vi "Navigation_Main_derping_stuff_up.vi"() -> ()   [LabVIEW 2015]
uses:
  <vilib>/myRIO/Instrument Drivers/Onboard IO/PWM/typedefs/PWM Reference.ctl
  <vilib>/myRIO/Common/Instrument Driver Framework/Utilities/typedefs/myRIO Generic Hardware Reference.ctl
  <vilib>/myRIO/Common/Instrument Driver Framework/Utilities/typedefs/Hardware Version Enum.ctl
  <vilib>/myRIO/Common/Instrument Driver Framework/Utilities/typedefs/myRIO v1.0 Reference.ctl
  <vilib>/myRIO/Common/Instrument Driver Framework/Utilities/typedefs/Generic FPGA Reference.ctl
  <vilib>/myRIO/Common/Instrument Driver Framework/myRIO v1.0/PWM/typedefs/PWM Channels Enum.ctl
  <vilib>/myRIO/Instrument Drivers/Onboard IO/PWM/typedefs/PWM Configuration.ctl
  <vilib>/userdefined/High Color/nirio_resource_hc.ctl
  <vilib>/myRIO/Common/Instrument Driver Framework/myRIO v1.0/PWM/vis/myRIO v1.1 Open PWM.vi
  <vilib>/myRIO/Common/Instrument Driver Framework/Utilities/vis/Validate Channels.vi
  <vilib>/myRIO/Common/Instrument Driver Framework/myRIO v1.0/PWM/vis/myRIO v1.0 Reserve PWM.vi
  <vilib>/myRIO/Common/Instrument Driver Framework/myRIO v1.0/PWM/vis/myRIO v1.0 Build MUX Configuration PWM.vi
  <vilib>/myRIO/Common/Instrument Driver Framework/myRIO v1.0/Resource Manager/vis/myRIO v1.0 Reserve Channel List.vi
  <vilib>/myRIO/Common/Instrument Driver Framework/myRIO v1.0/Resource Manager/vis/myRIO v1.0 Create Configuration List.vi
  <vilib>/myRIO/Common/Instrument Driver Framework/myRIO v1.0/Resource Manager/vis/myRIO v1.0 Reserve Channel.vi
  <vilib>/myRIO/Common/Instrument Driver Framework/myRIO v1.0/Resource Manager/vis/myRIO v1.0 Unreserve Channel.vi
  <vilib>/myRIO/Common/Instrument Driver Framework/myRIO v1.0/Resource Manager/vis/myRIO v1.0 Build Mutex Name.vi
  <vilib>/FPGAPlugInAG/myRIO-1900/niLvFpga_Open_myRIO-1900.vi
  <vilib>/rvi/interface/common/dynamic/niFpgaDynamicAddResources.vi
  <vilib>/myRIO/Common/Instrument Driver Framework/Utilities/vis/FPGA Ref Manager.vi
  <vilib>/Utility/error.llb/Error Cluster From Error Code.vi
  <vilib>/myRIO/Common/Instrument Driver Framework/Utilities/vis/Ref Counter.vi
  <vilib>/rvi/errors/niLvFpgaAdjustHostInterfaceError.vi
  <vilib>/Utility/VariantDataType/GetNumericInfo.vi
  <vilib>/myRIO/Common/Instrument Driver Framework/myRIO v1.0/myRIO v1.1 Open.vi
  <vilib>/myRIO/Common/Instrument Driver Framework/Utilities/vis/IO Manager.vi
  <vilib>/myRIO/Common/Instrument Driver Framework/Utilities/vis/Configuration Manager.vi
  <vilib>/myRIO/Common/Instrument Driver Framework/myRIO v1.0/Resource Manager/vis/myRIO v1.0 Configure IO.vi
  <vilib>/myRIO/Common/Instrument Driver Framework/myRIO v1.0/myRIO v1.0 Close.vi
  <vilib>/myRIO/Common/Instrument Driver Framework/myRIO v1.0/PWM/vis/myRIO v1.0 Write PWM.vi
  <vilib>/addons/control/pid/pid.llb/PID (DBL).vi
  <vilib>/rvi/interface/nirviOpenFPGA/nirviOpenFPGA.xnode
  Navi/E/FPGA Bitfiles/NavigationProjec_FPGATarget2_FPGAMainNavigati_PWPHW8gwDxI.lvbitx
  <vilib>/rvi/interface/nirviReadWriteControl/nirviReadWriteControl.xnode
  <vilib>/myRIO/Instrument Drivers/Onboard IO/PWM/vis/myRIO PWM Open.xnode
  <vilib>/myRIO/Instrument Drivers/Onboard IO/PWM/PWM.lvlib
  <vilib>/myRIO/Instrument Drivers/Utilities/Utilities.lvlib
  NiFpgaLv.dll
  <vilib>/rvi/interface/Simulation/niFpgaSimulationCallBeginRW.vi
  <vilib>/addons/control/pid/NI_PID_pid.lvlib
panel:
  out "goal reached":bool=TRUE
  out "x/y":dbl
  out "scale":dbl=1.0
  in  "x goal":dbl=10.0
  in  "L Desired Input Velocity (ft/s) 4":dbl(knob) scale=-4.0..4.0
  out "x position 5":dbl
  in  "R Min Linear Velocity (ft/s)  2":dbl=-2.0 format="%#_13g"
  in  "L Min Linear Velocity (ft/s) 9":dbl=-2.0 format="%#_13g"
  in  "R Max Linear Velocity (ft/s) 5":dbl=2.0 format="%#_13g"
  in  "L Max Linear Velocity (ft/s) 5":dbl=2.0 format="%#_13g"
  in  "R Desired Input Velocity (ft/s) 5":dbl(knob) scale=-4.0..4.0
  in  "R Desired Input Velocity (ft/s) 4":dbl(knob) scale=-4.0..4.0
  in  "L Desired Input Velocity (ft/s) 3":dbl(knob) scale=-4.0..4.0
  in  "R Desired Input Velocity (ft/s) 3":dbl(knob) scale=-4.0..4.0
  in  "L Desired Input Velocity (ft/s) 2":dbl(knob) scale=-4.0..4.0
  in  "R Desired Input Velocity (ft/s) 2":dbl(knob) scale=-4.0..4.0
  in  "L Desired Input Velocity (ft/s)":dbl(knob) scale=-4.0..4.0
  out "left":dbl
  out "right":dbl
  out "actual pwm 2":dbl
  in  "stop 3":bool
  out "left pwm":dbl(graph)
  out "dt out (s) 3":dbl format="%.3f"
  in  "output range 3":cluster{"output high":dbl, "output low":dbl}={"output high"=0.13333, "output low"=-0.13333} {"output low" format="%.6f"; "output high" format="%.5f"}
  in  "PID gains 3":T1={"proportional gain (Kc)"=0.002, "integral time (Ti, min)"=7e-07, "derivative time (Td, min)"=0.0} {"derivative time (Td, min)" format="%.8f"; "integral time (Ti, min)" format="%.8f"; "proportional gain (Kc)" format="%.8f"}
  out "desired pwm 2":dbl
  out "feedback 2":dbl
  out ".not. x? 3":bool
  out "Elapsed Time (s) 2":dbl caption="Elapsed Time (s)"
  out "x traveled 2":dbl
  out "y traveled 2":dbl
  out "avg 124":dbl
  out "avg 457":dbl
  out "psi dot 2":dbl
  out "distance traveled 2":dbl
  out "y dot 2":dbl
  out "x dot 2":dbl
  out "x position 2":dbl
  out "y position 2":dbl
  out "reset x y 2":dbl
  out "Tick Count(mSec) 2":u32 caption="Tick Count(mSec)"
  in  "start y 2":dbl=3.0
  in  "start x 2":dbl=1.0
  in  "Encoder Reset 3":bool
  out "ENC.B_c.CNTR 3":i32
  out "ENC.B_b.CNTR 3":i32
  out "ENC.B_a.CNTR 3":i32
  out "ENC.A_c.CNTR 3":i32
  out "ENC.A_b.CNTR 3":i32
  out "ENC.A_a.CNTR 3":i32
  in  "start y":dbl=3.0
  in  "start x":dbl=1.0
  in  "Encoder Reset 2":bool
  out "actual pwm":dbl
  in  "stop 2":bool
  out "right pwm":dbl(graph)
  out "dt out (s) 2":dbl format="%.3f"
  in  "output range 2":cluster{"output high":dbl, "output low":dbl}={"output high"=0.13333, "output low"=-0.13333} {"output low" format="%.6f"; "output high" format="%.5f"}
  in  "PID gains 2":T1={"proportional gain (Kc)"=0.002, "integral time (Ti, min)"=7e-07, "derivative time (Td, min)"=0.0} {"derivative time (Td, min)" format="%.8f"; "integral time (Ti, min)" format="%.8f"; "proportional gain (Kc)" format="%.8f"}
  out "desired pwm":dbl
  out "feedback":dbl
  out ".not. x? 2":bool
  out "Elapsed Time (s)":dbl
  out "LF Rot Velocity (rot/s)":dbl
  out "LM Rot Velocity (rot/s)":dbl
  out "LR Rot Velocity (rot/s)":dbl
  out "RR Rot Velocity (rot/s)":dbl
  out "RM Linear Velocity (rot/s)":dbl
  out "RF Linear Velocity (rot/s)":dbl
  in  "Encoder Reset":bool
  out "SYS.SELECTA":u8 format="%08b"
  out "ENC.B_c.CNTR":i32
  out "ENC.B_b.CNTR":i32
  out "ENC.B_a.CNTR":i32
  out "ENC.A_c.CNTR":i32
  out "ENC.A_b.CNTR":i32
  out "ENC.A_a.CNTR":i32
  in  "R Min Linear Velocity (ft/s)":dbl=-2.0 format="%#_13g"
  in  "R Max Linear Velocity (ft/s)":dbl=2.0 format="%#_13g"
  in  "L Min Linear Velocity (ft/s)":dbl=-2.0 format="%#_13g"
  in  "L Max Linear Velocity (ft/s)":dbl=2.0 format="%#_13g"
  out "Current Rot Velocity (rot/s)":T2(graph)
  # "Motor Control Parameters"
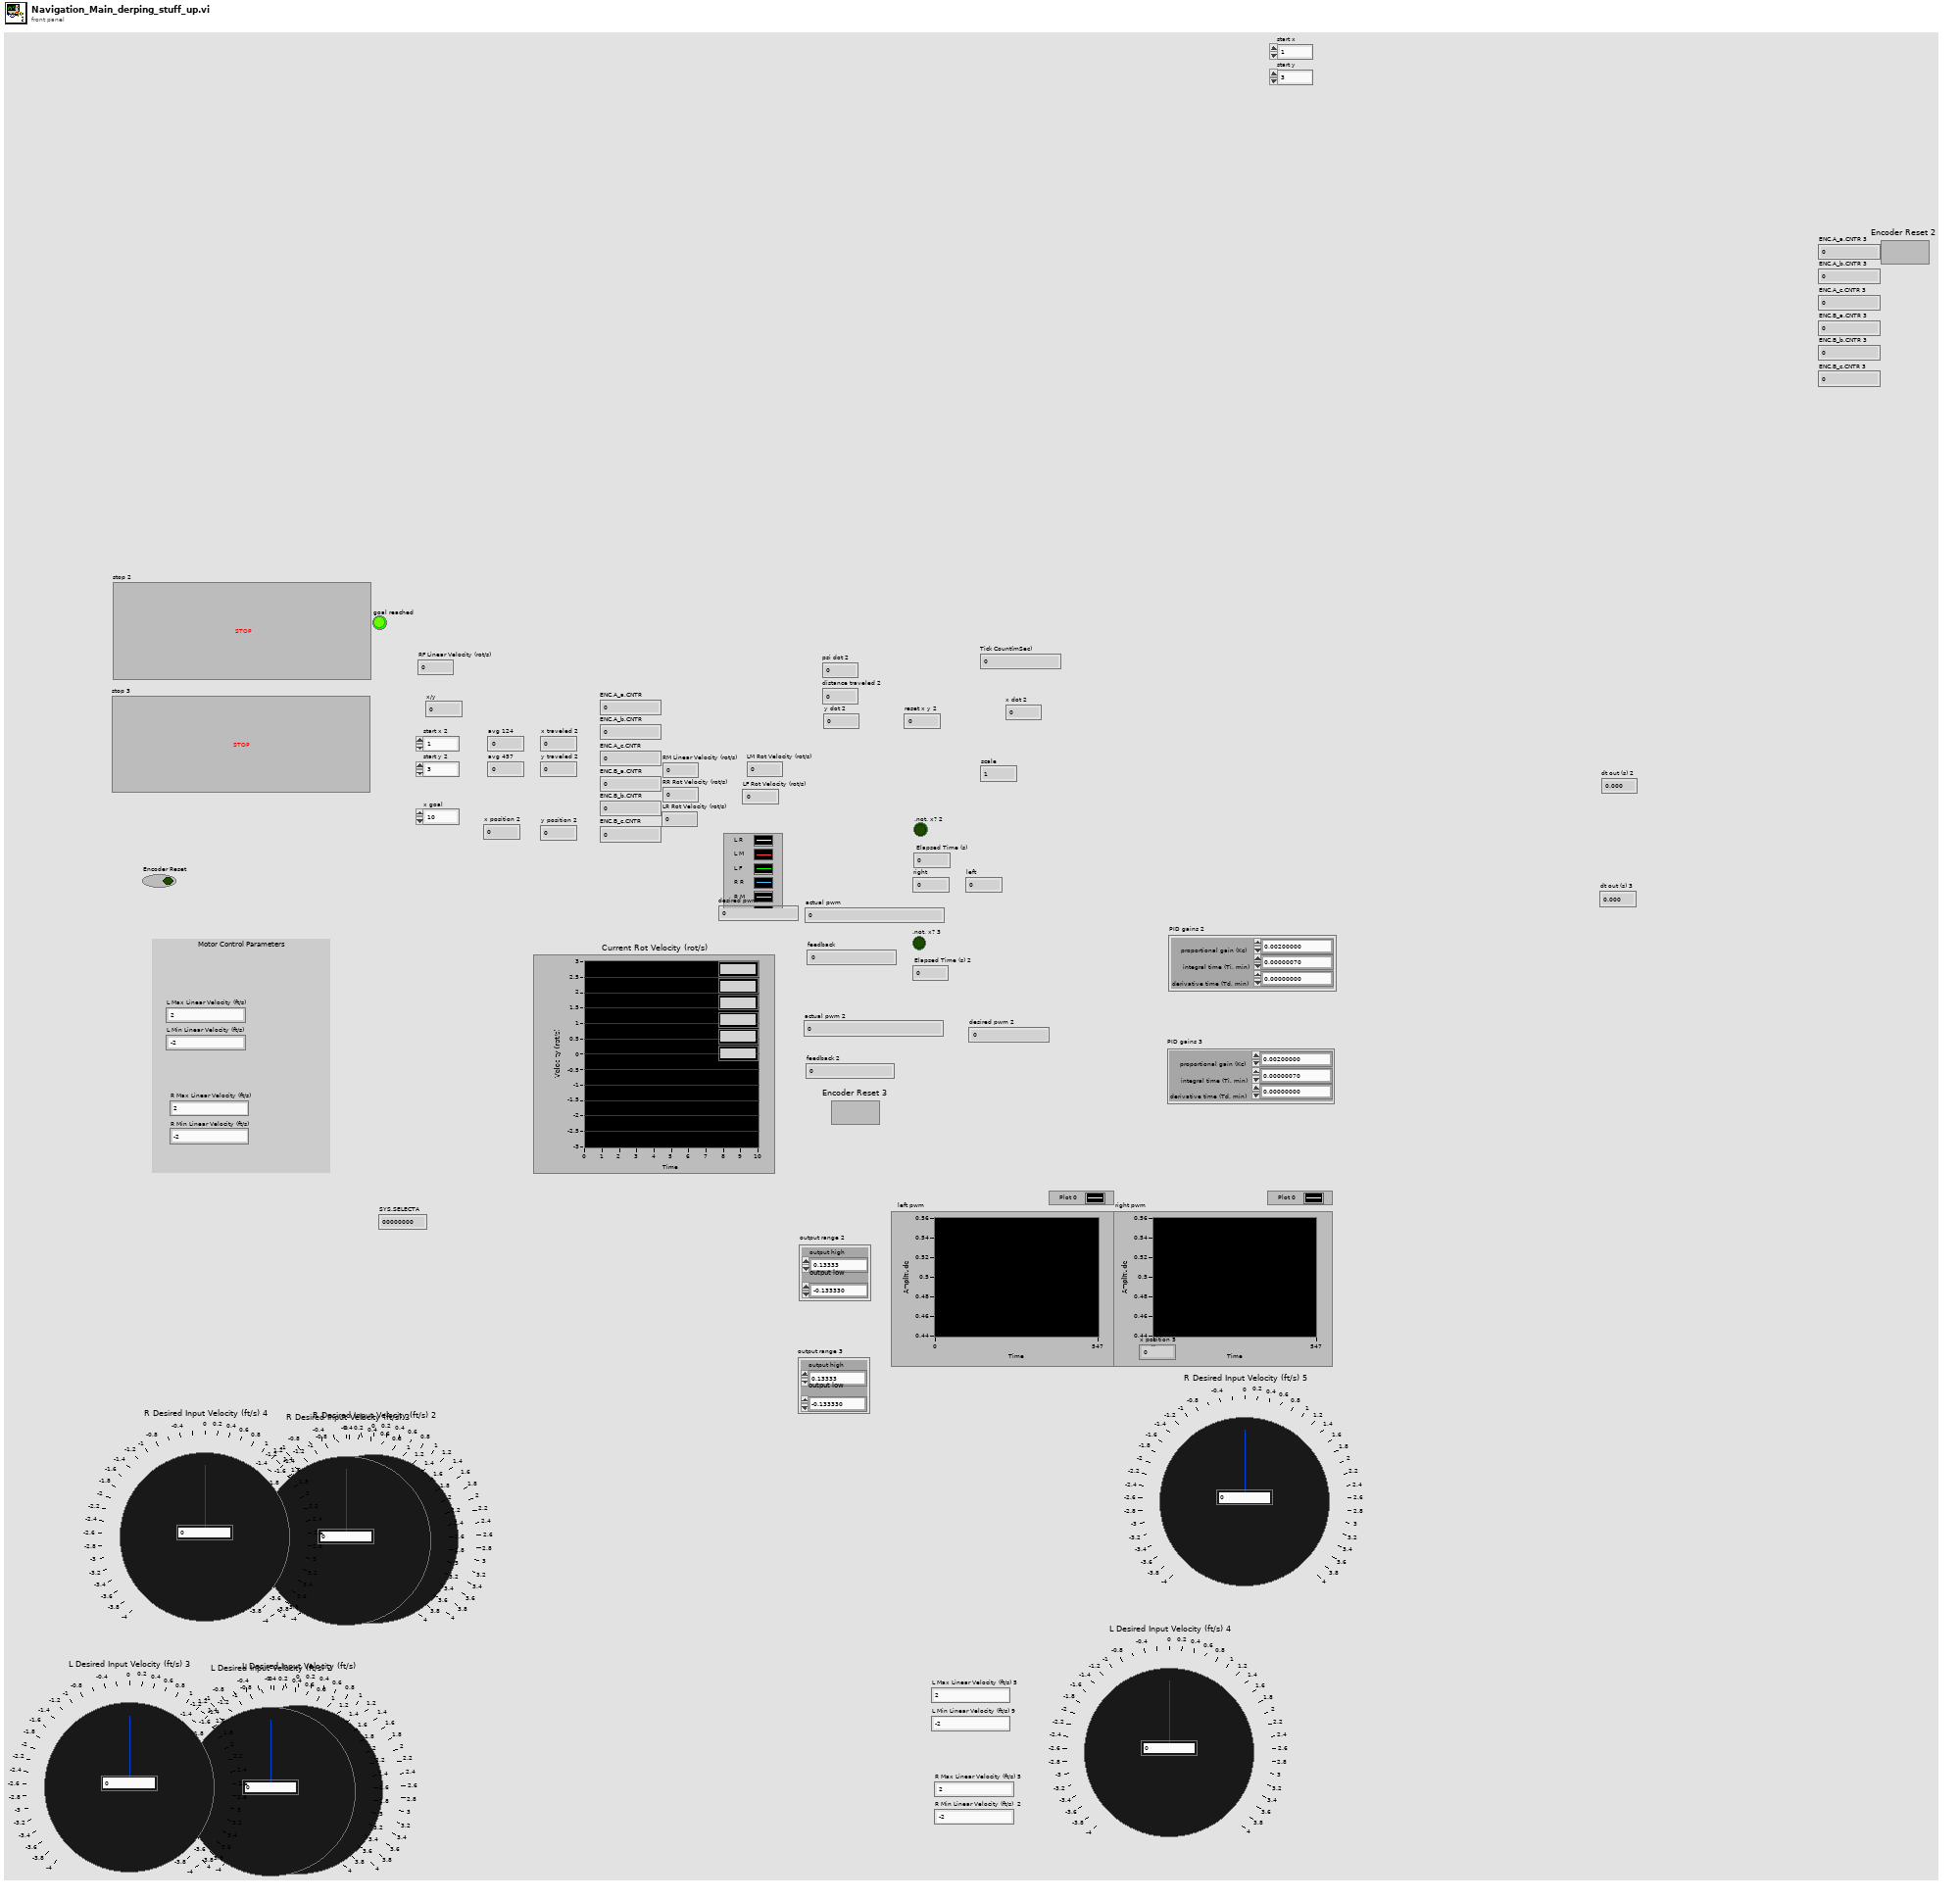
[diagram p1: front panel]
types:
  T1 = cluster{"proportional gain (Kc)":dbl, "integral time (Ti, min)":dbl, "derivative time (Td, min)":dbl}
  T2 = cluster{"Rotational Velocity (RPS)":dbl, "Rotational Velocity (RPS)":dbl, "Rotational Velocity (RPS)":dbl, "Rotational Velocity (RPS)":dbl, "Rotational Velocity (RPS)":dbl, "Rotational Velocity (RPS)":dbl}
  T3 = typedef "nirio_resource_hc.ctl" = tag
  T4 = typedef "Hardware Version Enum.ctl" = enum16{"Unknown", "myRIO-1900", "myRIO-1950", "roboRIO"}
  T5 = typedef "PWM.lvlib/PWM Reference.ctl" = cluster{"myRIO Reference":T6, "PWM Channels Enum":T9, "PWM Configuration":T10}
  T6 = typedef "myRIO Generic Hardware Reference.ctl" = cluster{"myRIO Model":T4, "myRIO Hardware Reference":T7}
  T7 = typedef "myRIO v1.0 Reference.ctl" = cluster{"Generic FPGA Reference":T8, "Allow multiple opens":bool}
  T8 = typedef "Generic FPGA Reference.ctl" = refnum<k20>
  T9 = typedef "PWM Channels Enum.ctl" = enum16{"Not Connected", "C/PWM0", "C/PWM1", "A/PWM0", "A/PWM1", "A/PWM2", "B/PWM0", "B/PWM1", "B/PWM2", "PWM/PWM0", "PWM/PWM1", "PWM/PWM2", "PWM/PWM3", "PWM/PWM4", "PWM/PWM5", "PWM/PWM6", "PWM/PWM7", "PWM/PWM8", "PWM/PWM9"}
  T10 = typedef "PWM.lvlib/PWM Configuration.ctl" = cluster{"Frequency":dbl, "Duty Cycle":dbl}
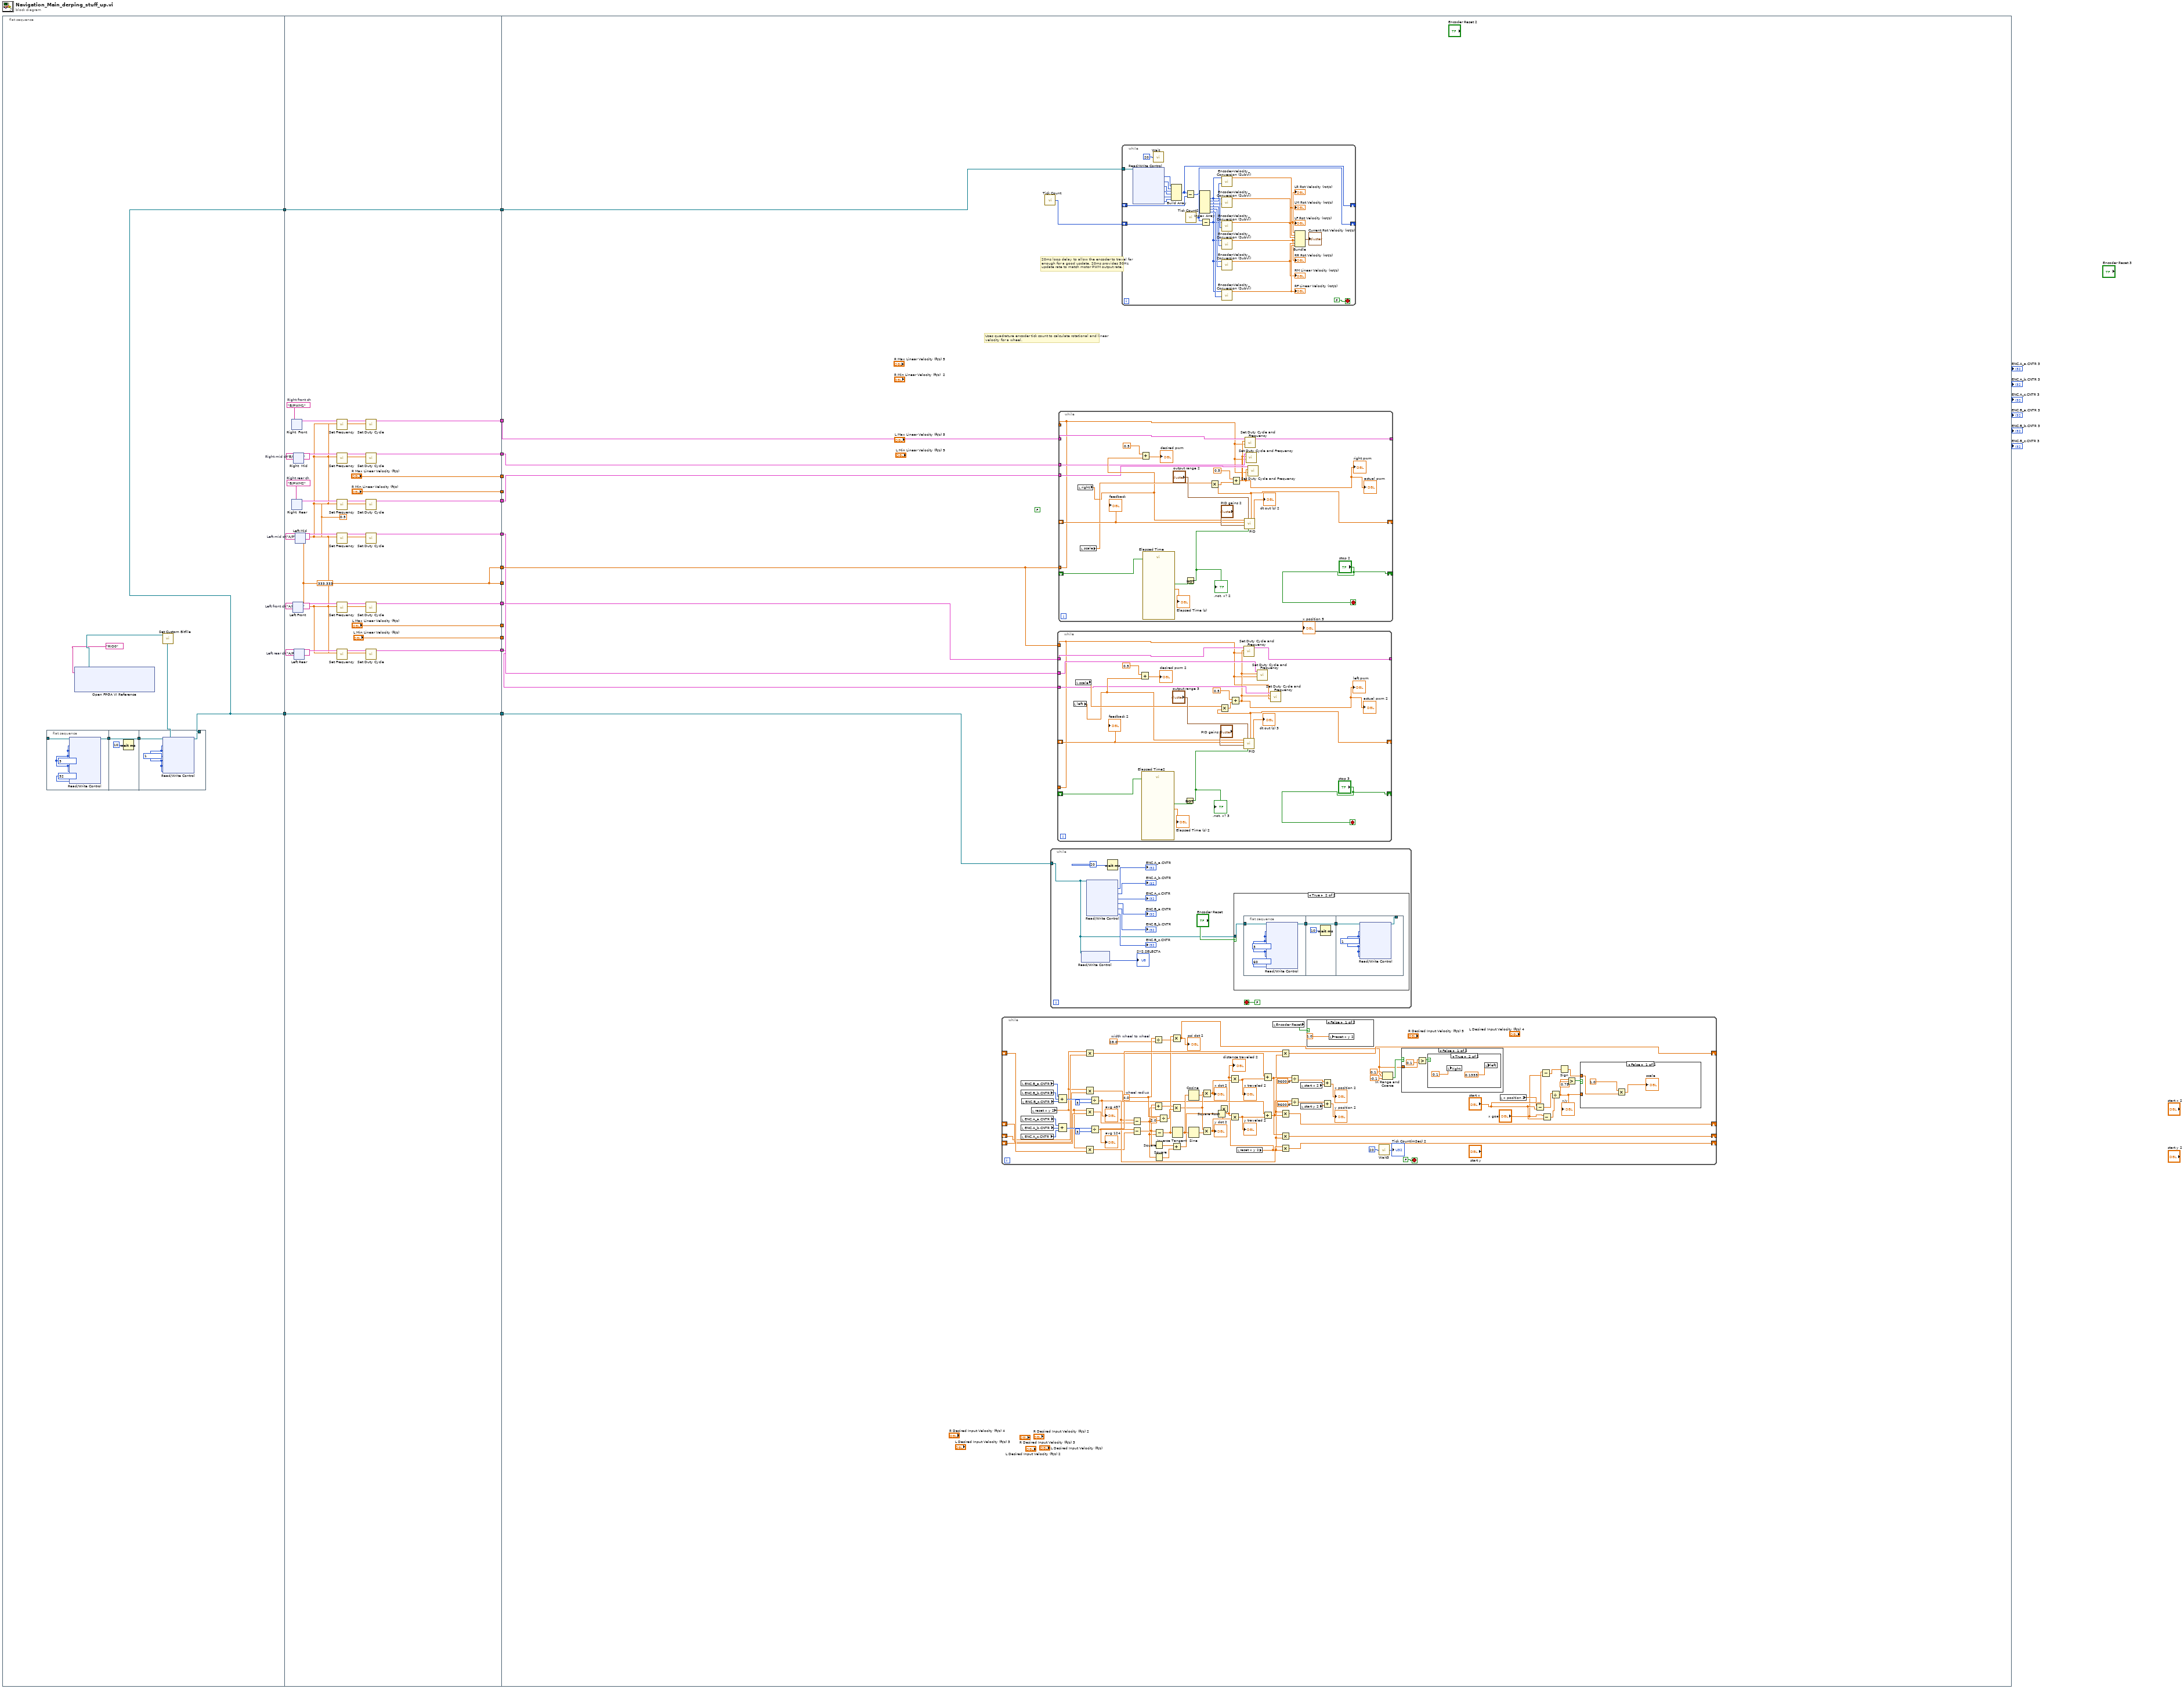
[diagram p0: block diagram]
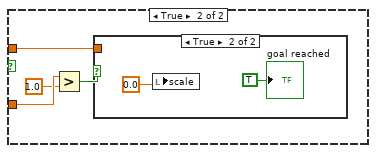
[diagram p2: hidden frame]
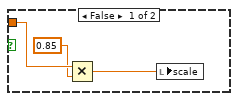
[diagram p3: hidden frame]
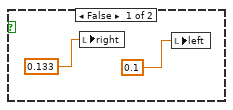
[diagram p4: hidden frame]
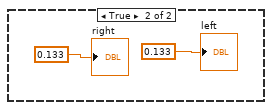
[diagram p5: hidden frame]
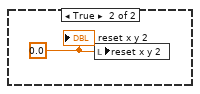
[diagram p6: hidden frame]
diagram:
  n1 = flat-sequence {
    tunnel: [w19] -> w4
    tunnel: [w19] -> w2
    tunnel: [w32] -> w16
    tunnel: [w47] -> w15
    tunnel: [w43] -> w14
    tunnel: [w42] -> w13
    tunnel: [w41] -> w12
    tunnel: [w40] -> w11
    tunnel: [w39] -> w10
    tunnel: ["L Max Linear Velocity (ft/s)"] -> w9
    tunnel: ["L Min Linear Velocity (ft/s)"] -> w8
    tunnel: ["R Max Linear Velocity (ft/s)"] -> w7
    tunnel: ["R Min Linear Velocity (ft/s)"] -> w6
    tunnel: [w34] -> w5
    tunnel: w4 -> [w33]
    tunnel: [w33] -> w3
    tunnel: w2 -> [w34]
    tunnel: [w32] -> w1
    tunnel: w16 -> [_]
    tunnel: w15 -> [w160]
    tunnel: w14 -> [w166]
    tunnel: w13 -> [w163]
    tunnel: w12 -> [w162]
    tunnel: w11 -> [w161]
    tunnel: w10 -> [w165]
    tunnel: w9 -> [_]
    tunnel: w8 -> [_]
    tunnel: w7 -> [_]
    tunnel: w6 -> [_]
    tunnel: w5 -> [w168]
    tunnel: w3 -> [w167]
    tunnel: w1 -> [w164]
    frame #0 {
      n2 = flat-sequence {
        tunnel: w20 -> [w25]
        tunnel: [w23] -> w22
        tunnel: w22 -> [w27]
        tunnel: [w27] -> w21
        tunnel: w21 -> [w30]
        tunnel: [w29] -> w19
        frame #0 {
          w24 = u8 32 ("SYS.SELECTA")
          w26 = u8 3 ("ENC.B_c.CNFG")
          n3 = xnode "Read/Write Control"("FPGA VI Reference In"=w25, "ENC.A_a.CNFG"=w26, "ENC.A_b.CNFG"=w26, "ENC.A_c.CNFG"=w26, "ENC.B_a.CNFG"=w26, "ENC.B_b.CNFG"=w26, "ENC.B_c.CNFG"=w26, "SYS.SELECTA"=w24, "SYS.SELECTB"=w24) -> ("FPGA VI Reference Out"=w23:refnum<k20>)  [unwired: 1 in, 1 out]
        }
        frame #1 {
          n4 = Wait (ms)(milliseconds to wait=u32 10) -> ()  [unwired: 1 out]
        }
        frame #2 {
          w31 = u8 1 ("ENC.B_c.CNFG")
          n5 = xnode "Read/Write Control"("FPGA VI Reference In"=w30, "ENC.A_a.CNFG"=w31, "ENC.A_b.CNFG"=w31, "ENC.A_c.CNFG"=w31, "ENC.B_a.CNFG"=w31, "ENC.B_b.CNFG"=w31, "ENC.B_c.CNFG"=w31) -> ("FPGA VI Reference Out"=w29:refnum<k20>)  [unwired: 1 in, 1 out]
        }
      }
      n6 = xnode "Open FPGA VI Reference"("resource name"=tag "RIO0") -> ("FPGA VI Reference Out"=w18:refnum<k20>)  [unwired: 1 in, 1 out]
      n7 = call <vilib>:"Set Custom Bitfile.vi"("Custom FPGA Reference In"=w18) -> ("Custom FPGA Reference Out"=w20:refnum<k20>)  [unwired: 9 in, 1 out]
    }
    frame #1 {
      w44 = 0.5 ("Duty Cycle")
      w32 = 333.333 ("Frequency [Hz]")
      w58 = tag "B/PWM2"  # Right rear ch
      w59 = tag "B/PWM0"  # Right mid ch
      w60 = tag "B/PWM1"  # Right front ch
      w61 = tag "A/PWM2"  # Left rear ch
      w62 = tag "A/PWM1"  # Left mid ch
      w63 = tag "A/PWM0"  # Left front ch
      n8 = xnode "Right  Front"("Channel Name"=w60) -> ("PWM Ref Out"=w54:T5)  [unwired: 2 in, 1 out]
      n9 = xnode "Right  Rear"("Channel Name"=w58) -> ("PWM Ref Out"=w52:T5)  [unwired: 2 in, 1 out]
      n10 = xnode "Left Front"("Channel Name"=w63) -> ("PWM Ref Out"=w57:T5)  [unwired: 2 in, 1 out]
      n11 = xnode "Right  Mid"("Channel Name"=w59) -> ("PWM Ref Out"=w53:T5)  [unwired: 2 in, 1 out]
      n12 = xnode "Left Rear"("Channel Name"=w61) -> ("PWM Ref Out"=w55:T5)  [unwired: 2 in, 1 out]
      n13 = xnode "Left Mid"("Channel Name"=w62) -> ("PWM Ref Out"=w56:T5)  [unwired: 2 in, 1 out]
      n14 = call <vilib>:"Set Frequency.vi"("Frequency [Hz]"=w32, "PWM Ref In"=w54) -> ("PWM Ref Out"=w48:T5)  [unwired: 7 in, 1 out]
      n15 = call <vilib>:"Set Frequency.vi"("Frequency [Hz]"=w32, "PWM Ref In"=w53) -> ("PWM Ref Out"=w49:T5)  [unwired: 7 in, 1 out]
      n16 = call <vilib>:"Set Frequency.vi"("Frequency [Hz]"=w32, "PWM Ref In"=w52) -> ("PWM Ref Out"=w50:T5)  [unwired: 7 in, 1 out]
      n17 = call <vilib>:"Set Frequency.vi"("Frequency [Hz]"=w32, "PWM Ref In"=w56) -> ("PWM Ref Out"=w45:T5)  [unwired: 7 in, 1 out]
      n18 = call <vilib>:"Set Frequency.vi"("Frequency [Hz]"=w32, "PWM Ref In"=w57) -> ("PWM Ref Out"=w51:T5)  [unwired: 7 in, 1 out]
      n19 = call <vilib>:"Set Frequency.vi"("Frequency [Hz]"=w32, "PWM Ref In"=w55) -> ("PWM Ref Out"=w46:T5)  [unwired: 7 in, 1 out]
      n20 = call <vilib>:"Set Duty Cycle.vi"("Duty Cycle"=w44, "PWM Ref In"=w48) -> ("PWM Ref Out"=w43:T5)  [unwired: 7 in, 1 out]
      n21 = call <vilib>:"Set Duty Cycle.vi"("Duty Cycle"=w44, "PWM Ref In"=w49) -> ("PWM Ref Out"=w42:T5)  [unwired: 7 in, 1 out]
      n22 = call <vilib>:"Set Duty Cycle.vi"("Duty Cycle"=w44, "PWM Ref In"=w50) -> ("PWM Ref Out"=w41:T5)  [unwired: 7 in, 1 out]
      n23 = call <vilib>:"Set Duty Cycle.vi"("Duty Cycle"=w44, "PWM Ref In"=w45) -> ("PWM Ref Out"=w40:T5)  [unwired: 7 in, 1 out]
      n24 = call <vilib>:"Set Duty Cycle.vi"("Duty Cycle"=w44, "PWM Ref In"=w51) -> ("PWM Ref Out"=w39:T5)  [unwired: 7 in, 1 out]
      n25 = call <vilib>:"Set Duty Cycle.vi"("Duty Cycle"=w44, "PWM Ref In"=w46) -> ("PWM Ref Out"=w47:T5)  [unwired: 7 in, 1 out]
    }
    frame #2 {
      (unwired) FALSE
      # "Uses quadrature encoder tick count to calculate rotational and linear velocity for a wheel."
      # "20ms loop delay to allow the encoder to travel far enough for a good update. 20ms provides 50Hz update rate to match motor PWM output rate."
      n26 = while {
        shift-right: [w216] -> _
        shift-left: _ -> [w254]
        shift-right: [w213] -> _
        shift-left: _ -> [w253]
        shift-right: [w215] -> _
        shift-left: _ -> [w228]
        shift-right: [w214] -> _
        shift-left: _ -> [w227]
        stop <- FALSE stop-if-true
        w249 = 28.0  # width wheel to wheel
        w250 = 4.0  # wheel radius
        n27 = local read "ENC.B_a.CNTR"() -> (w259:i32)
        n28 = local read "ENC.B_b.CNTR"() -> (w258:i32)
        n29 = local read "ENC.A_a.CNTR"() -> (w262:i32)
        n30 = local read "ENC.A_b.CNTR"() -> (w261:i32)
        n31 = local read "ENC.A_c.CNTR"() -> (w260:i32)
        n32 = local read "ENC.B_c.CNTR"() -> (w257:i32)
        n33 = local read "reset x y 2"() -> (w212:dbl)
        n34 = Compound Arithmetic op=ADD(w259, w258, w257) -> (w265:i32)
        n35 = Compound Arithmetic op=ADD(w262, w261, w260) -> (w266:i32)
        n36 = Multiply(x=w212, y=w227) -> (x*y=w218:dbl)
        n37 = Multiply(x=w212, y=w228) -> (x*y=w219:dbl)
        n38 = Multiply(x=w212, y=w253) -> (x*y=w217:dbl)
        n39 = Multiply(x=w212, y=w254) -> (x*y=w220:dbl)
        n40 = Divide(x=w265, y=3) -> (x/y=w252:dbl)
        "avg 457" <- w252
        n41 = Divide(x=w266, y=3) -> (x/y=w255:dbl)
        "avg 124" <- w255
        n42 = Subtract(x=w252, y=w217) -> (x-y=w242:dbl)
        n43 = Subtract(x=w255, y=w220) -> (x-y=w243:dbl)
        n44 = Divide(x=w250, y=w249) -> (x/y=w245:dbl)
        n45 = Add(x=w243, y=w242) -> (x+y=w247:dbl)
        n46 = Square(x=w243) -> (x^2=w240:dbl)
        n47 = Square(x=w242) -> (x^2=w241:dbl)
        n48 = Subtract(x=w243, y=w242) -> (x-y=w246:dbl)
        n49 = Divide(x=w250, y=2.0) -> (x/y=w248:dbl)
        n50 = Multiply(x=w246, y=w245) -> (x*y=w202:dbl)
        "psi dot 2" <- w202
        n51 = Multiply(x=w247, y=w248) -> (x*y=w236:dbl)
        n52 = Add(x=w240, y=w241) -> (x+y=w239:dbl)
        n53 = Inverse Tangent(1:w246) -> (0:w244:dbl)
        n54 = Cosine(x=w244) -> (cos(x)=w237:dbl)
        n55 = Sine(x=w244) -> (sin(x)=w238:dbl)
        n56 = Multiply(x=w236, y=w237) -> (x*y=w234:dbl)
        "x dot 2" <- w234
        n57 = Multiply(x=w236, y=w238) -> (x*y=w235:dbl)
        "y dot 2" <- w235
        n58 = Square Root(x=w239) -> (sqrt(x)=w233:dbl)
        n59 = local read "reset x y 2"() -> (w210:dbl)
        n60 = Multiply(x=w233, y=w210) -> (x*y=w211:dbl)
        "distance traveled 2" <- w211
        n61 = Multiply(x=w211, y=w234) -> (x*y=w232:dbl)
        "x traveled 2" <- w232
        n62 = Multiply(x=w211, y=w235) -> (x*y=w231:dbl)
        "y traveled 2" <- w231
        n63 = Add(x=w218, y=w232) -> (x+y=w230:dbl)
        n64 = Add(x=w219, y=w231) -> (x+y=w222:dbl)
        n65 = local read "Encoder Reset"() -> (w209:bool)
        n66 = Multiply(x=w255, y=w210) -> (x*y=w216:dbl)
        n67 = Multiply(x=w210, y=w222) -> (x*y=w215:dbl)
        n68 = Multiply(x=w230, y=w210) -> (x*y=w214:dbl)
        n69 = Multiply(x=w252, y=w210) -> (x*y=w213:dbl)
        n70 = Divide(x=w230, y=9600.0) -> (x/y=w225:dbl)
        n71 = Divide(x=w222, y=9600.0) -> (x/y=w226:dbl)
        n72 = local read "start x 2"() -> (w223:dbl)
        n73 = local read "start y 2"() -> (w224:dbl)
        n74 = case shown="False" w209 {
          frame False {
            n75 = local write "reset x y 2"(1.0) -> ()
          }
          frame True {
            w290 = 0.0
            n76 = local write "reset x y 2"(w290) -> ()
            "reset x y 2" <- w290
          }
        }
        n77 = Add(x=w225, y=w223) -> (x+y=→"x position 2":dbl)
        n78 = Add(x=w226, y=w224) -> (x+y=→"y position 2":dbl)
        n79 = call "Wait3"("Count(mSec)"=u32 20) -> ("Tick Count(mSec)"=→"Tick Count(mSec) 2":u32)
        n80 = In Range and Coerce(upper limit=0.1, x=w202, lower limit=-0.1) -> (In Range?=w203:bool)  [unwired: 1 out]
        n81 = case shown="False" w203 {
          tunnel: w202 -> [w282 _]
          frame False {
            n82 = Greater?(x=w282, y=0.1) -> (0:w280:bool)
            n83 = case shown="True" w280 {
              frame False {
                n84 = local write "right"(0.133) -> ()
                n85 = local write "left"(0.1) -> ()
              }
              frame True {
                n86 = local write "right"(0.1) -> ()
                n87 = local write "left"(0.1333) -> ()
              }
            }
          }
          frame True {
            "right" <- 0.133
            "left" <- 0.133
          }
        }
        n88 = local read "x position 2"() -> (w201:dbl)
        n89 = Subtract(x=w201, y="start x") -> (x-y=w197:dbl)
        n90 = Subtract(x="start x", y="x goal") -> (x-y=w193:dbl)
        n91 = Subtract(x="x goal", y="start x") -> (x-y=w196:dbl)
        n92 = Divide(x=w197, y=w196) -> (x/y=w198:dbl)
        "x/y" <- w198
        n93 = Sign(1:w193) -> (0:w192:dbl)
        n94 = Greater?(x=w198, y=0.75) -> (0:w199:bool)
        n95 = case shown="False" w199 {
          tunnel: w198 -> [_ w274]
          tunnel: w192 -> [w269 w271]
          frame False {
            n96 = Multiply(x=1.0, y=w269) -> (x*y=→"scale":dbl)
          }
          frame True {
            n97 = Greater?(x=w274, y=1.0) -> (0:w272:bool)
            n98 = case shown="True" w272 {
              tunnel: w271 -> [w277 _]
              frame False {
                n99 = Multiply(x=w277, y=0.85) -> (x*y=w275:dbl)
                n100 = local write "scale"(w275) -> ()
              }
              frame True {
                n101 = local write "scale"(0.0) -> ()
                "goal reached" <- TRUE
              }
            }
          }
        }
      }
      n102 = call "Tick Count"() -> ("Tick Count(uSec)"=w169:u32)
      n103 = while {
        tunnel: w168 -> [w313]
        stop <- FALSE stop-if-true
        n104 = xnode "Read/Write Control"("FPGA VI Reference In"=w313) -> ("SYS.SELECTA"=→"SYS.SELECTA":u8)  [unwired: 1 in, 2 out]
        n105 = xnode "Read/Write Control"("FPGA VI Reference In"=w313) -> ("ENC.A_a.CNTR"=→"ENC.A_a.CNTR":u32, "ENC.A_b.CNTR"=→"ENC.A_b.CNTR":u32, "ENC.A_c.CNTR"=→"ENC.A_c.CNTR":u32, "ENC.B_a.CNTR"=→"ENC.B_a.CNTR":u32, "ENC.B_b.CNTR"=→"ENC.B_b.CNTR":u32, "ENC.B_c.CNTR"=→"ENC.B_c.CNTR":u32)  [unwired: 1 in, 2 out]
        n106 = Wait (ms)(milliseconds to wait=u32 20) -> ()  [unwired: 1 out]
        n107 = case shown="True" "Encoder Reset" {
          tunnel: w313 -> [_ w324]
          frame False {
          }
          frame True {
            n108 = flat-sequence {
              tunnel: w324 -> [w329]
              tunnel: [w327] -> w326
              tunnel: w326 -> [w331]
              tunnel: [w331] -> w325
              tunnel: w325 -> [w334]
              tunnel: [w333] -> _
              frame #0 {
                w328 = u8 60 ("SYS.SELECTA")
                w330 = u8 3 ("ENC.B_c.CNFG")
                n109 = xnode "Read/Write Control"("FPGA VI Reference In"=w329, "ENC.A_a.CNFG"=w330, "ENC.A_b.CNFG"=w330, "ENC.A_c.CNFG"=w330, "ENC.B_a.CNFG"=w330, "ENC.B_b.CNFG"=w330, "ENC.B_c.CNFG"=w330, "SYS.SELECTA"=w328, "SYS.SELECTB"=w328) -> ("FPGA VI Reference Out"=w327:refnum<k20>)  [unwired: 1 in, 1 out]
              }
              frame #1 {
                n110 = Wait (ms)(milliseconds to wait=u32 10) -> ()  [unwired: 1 out]
              }
              frame #2 {
                w335 = u8 1 ("ENC.B_c.CNFG")
                n111 = xnode "Read/Write Control"("FPGA VI Reference In"=w334, "ENC.A_a.CNFG"=w335, "ENC.A_b.CNFG"=w335, "ENC.A_c.CNFG"=w335, "ENC.B_a.CNFG"=w335, "ENC.B_b.CNFG"=w335, "ENC.B_c.CNFG"=w335) -> ("FPGA VI Reference Out"=w333:refnum<k20>)  [unwired: 1 in, 1 out]
              }
            }
          }
        }
      }
      n112 = while {
        tunnel: w165 -> [w190]
        tunnel: [w191] -> _
        tunnel: w164 -> [w170]
        shift-right: [w176] -> _
        shift-left: _ -> [w186]
        shift-right: ["stop 3"] -> _
        shift-left: _ -> [w181]
        tunnel: [w170] -> _
        tunnel: w161 -> [w173]
        tunnel: w160 -> [w172]
        stop <- "stop 3" stop-if-true
        n113 = local read "left"() -> (w174:dbl)
        n114 = local read "scale"() -> (w177:dbl)
        n115 = Add(x=0.5, y=w174) -> (x+y=→"desired pwm 2":dbl)
        n116 = call "Elapsed Time2"("Reset"=w181) -> ("Elapsed Time (s)"=→"Elapsed Time (s) 2":dbl, "Time has Elapsed"=w184:bool)  [unwired: 11 in, 6 out]
        n117 = Not(x=w184) -> (.not. x?=w183:bool)
        ".not. x? 3" <- w183
        n118 = call-poly <vilib>:"PID.vi"("reinitialize? (F)"=w183, "output range"="output range 3", "PID gains"="PID gains 3", "process variable"=w186, "setpoint"=w174) -> ("dt out (s)"=→"dt out (s) 3":dbl, "output"=w176:dbl)  [unwired: 5 in]
        n119 = Multiply(x=w177, y=w176) -> (x*y=w175:dbl)
        n120 = Add(x=0.5, y=w175) -> (x+y=w171:dbl)
        "actual pwm 2" <- w171
        "left pwm" <- w171
        n121 = call <vilib>:"Set Duty Cycle and Frequency.vi"("Frequency [Hz]"=w170, "Duty Cycle"=w171, "PWM Ref In"=w190) -> ("PWM Ref Out"=w191:T5)  [unwired: 6 in, 1 out]
        n122 = call <vilib>:"Set Duty Cycle and Frequency.vi"("Frequency [Hz]"=w170, "Duty Cycle"=w171, "PWM Ref In"=w173) -> ()  [unwired: 6 in, 2 out]
        n123 = call <vilib>:"Set Duty Cycle and Frequency.vi"("Frequency [Hz]"=w170, "Duty Cycle"=w171, "PWM Ref In"=w172) -> ()  [unwired: 6 in, 2 out]
        "feedback 2" <- w186
      }
      n124 = while {
        tunnel: w166 -> [w311]
        tunnel: [w312] -> _
        tunnel: [w291] -> _
        shift-right: [w297] -> _
        shift-left: _ -> [w307]
        shift-right: ["stop 2"] -> _
        shift-left: _ -> [w302]
        tunnel: w164 -> [w291]
        tunnel: w163 -> [w294]
        tunnel: w162 -> [w293]
        stop <- "stop 2" stop-if-true
        n125 = local read "right"() -> (w295:dbl)
        n126 = local read "scale"() -> (w298:dbl)
        n127 = Add(x=0.5, y=w295) -> (x+y=→"desired pwm":dbl)
        n128 = call "Elapsed Time"("Reset"=w302) -> ("Elapsed Time (s)"=→"Elapsed Time (s)":dbl, "Time has Elapsed"=w305:bool)  [unwired: 11 in, 6 out]
        n129 = Not(x=w305) -> (.not. x?=w304:bool)
        ".not. x? 2" <- w304
        n130 = call-poly <vilib>:"PID.vi"("reinitialize? (F)"=w304, "output range"="output range 2", "PID gains"="PID gains 2", "process variable"=w307, "setpoint"=w295) -> ("dt out (s)"=→"dt out (s) 2":dbl, "output"=w297:dbl)  [unwired: 5 in]
        n131 = Multiply(x=w298, y=w297) -> (x*y=w296:dbl)
        n132 = Add(x=0.5, y=w296) -> (x+y=w292:dbl)
        "actual pwm" <- w292
        "right pwm" <- w292
        n133 = call <vilib>:"Set Duty Cycle and Frequency.vi"("Frequency [Hz]"=w291, "Duty Cycle"=w292, "PWM Ref In"=w311) -> ("PWM Ref Out"=w312:T5)  [unwired: 6 in, 1 out]
        n134 = call <vilib>:"Set Duty Cycle and Frequency.vi"("Frequency [Hz]"=w291, "Duty Cycle"=w292, "PWM Ref In"=w294) -> ()  [unwired: 6 in, 2 out]
        n135 = call <vilib>:"Set Duty Cycle and Frequency.vi"("Frequency [Hz]"=w291, "Duty Cycle"=w292, "PWM Ref In"=w293) -> ()  [unwired: 6 in, 2 out]
        "feedback" <- w307
      }
      n136 = while {
        shift-right: [w354] -> _
        shift-left: _ -> [w353]
        shift-right: [w351] -> _
        shift-left: w169 -> [w350]
        tunnel: w167 -> [w361]
        stop <- FALSE stop-if-true
        n137 = xnode "Read/Write Control"("FPGA VI Reference In"=w361) -> ("ENC.A_a.CNTR"=w360:u32, "ENC.A_b.CNTR"=w359:u32, "ENC.A_c.CNTR"=w358:u32, "ENC.B_a.CNTR"=w357:u32, "ENC.B_b.CNTR"=w356:u32, "ENC.B_c.CNTR"=w355:u32)  [unwired: 1 in, 2 out]
        n138 = call "Wait"("Count(mSec)"=u32 20) -> ()  [unwired: 1 out]
        n139 = Build Array(w360, w359, w358, w357, w356, w355) -> (w354:u32[])
        n140 = Subtract(x=w354, y=w353) -> (x-y=w352:u32[])
        n141 = call "Tick Count2"() -> ("Tick Count(uSec)"=w351:u32)
        n142 = Index Array(array=w352) -> (element #1=w349:u32, element #2=w348:u32, element #3=w347:u32, element #4=w346:u32, element #5=w345:u32, element #6=w344:u32)  [unwired: 6 in]
        n143 = Subtract(x=w351, y=w350) -> (x-y=w343:u32)
        n144 = call "Encoder-Velocity_Conversion (SubVI).vi"("delta  Encoder Count"=w348, "dt (uSec)"=w343) -> ("Rotational Velocity (RPS)"=w338:dbl)  [unwired: 7 in, 2 out]
        "LM Rot Velocity (rot/s)" <- w338
        n145 = call "Encoder-Velocity_Conversion (SubVI).vi"("delta  Encoder Count"=w347, "dt (uSec)"=w343) -> ("Rotational Velocity (RPS)"=w337:dbl)  [unwired: 7 in, 2 out]
        "LF Rot Velocity (rot/s)" <- w337
        n146 = call "Encoder-Velocity_Conversion (SubVI).vi"("delta  Encoder Count"=w349, "dt (uSec)"=w343) -> ("Rotational Velocity (RPS)"=w339:dbl)  [unwired: 7 in, 2 out]
        "LR Rot Velocity (rot/s)" <- w339
        n147 = call "Encoder-Velocity_Conversion (SubVI).vi"("delta  Encoder Count"=w346, "dt (uSec)"=w343) -> ("Rotational Velocity (RPS)"=w336:dbl)  [unwired: 7 in, 2 out]
        "RR Rot Velocity (rot/s)" <- w336
        n148 = call "Encoder-Velocity_Conversion (SubVI).vi"("delta  Encoder Count"=w345, "dt (uSec)"=w343) -> ("Rotational Velocity (RPS)"=w340:dbl)  [unwired: 7 in, 2 out]
        "RM Linear Velocity (rot/s)" <- w340
        n149 = call "Encoder-Velocity_Conversion (SubVI).vi"("delta  Encoder Count"=w344, "dt (uSec)"=w343) -> ("Rotational Velocity (RPS)"=w341:dbl)  [unwired: 7 in, 2 out]
        "RF Linear Velocity (rot/s)" <- w341
        n150 = Bundle("Rotational Velocity (RPS)"=w339, "Rotational Velocity (RPS)"=w338, "Rotational Velocity (RPS)"=w337, "Rotational Velocity (RPS)"=w336, "Rotational Velocity (RPS)"=w340, "Rotational Velocity (RPS)"=w341) -> (→"Current Rot Velocity (rot/s)":T2)  [unwired: 1 in]
      }
    }
  }
